vi "ToolBarcode (Get).vi"(7 "LabVIEW Web Service Request":refnum<class "Web Request.lvclass">) -> ()   [LabVIEW 2019]
uses:
  <vilib>/wsapi/Web Request.lvclass
  QDMH support files/QDMH Poly VIs/QDMH POLY Enqueue String.vi
panel:
  # "Use the Web Service Request input terminal to call the VIs on the Web Services palette. Do not remove it from the connector pane unless you don't need access to the palette."
  # "Each additional control wired to the connector pane will be available as an input in the URL. To include an indicator in terminal-mode output (the default setting), it must also be wired to the connector pane."
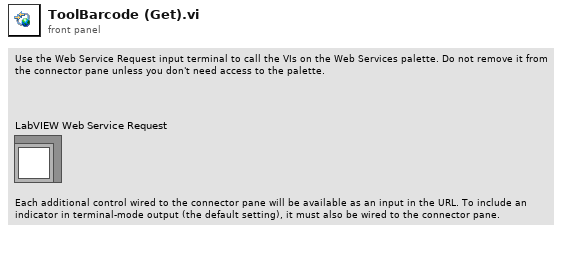
[diagram p1: front panel]
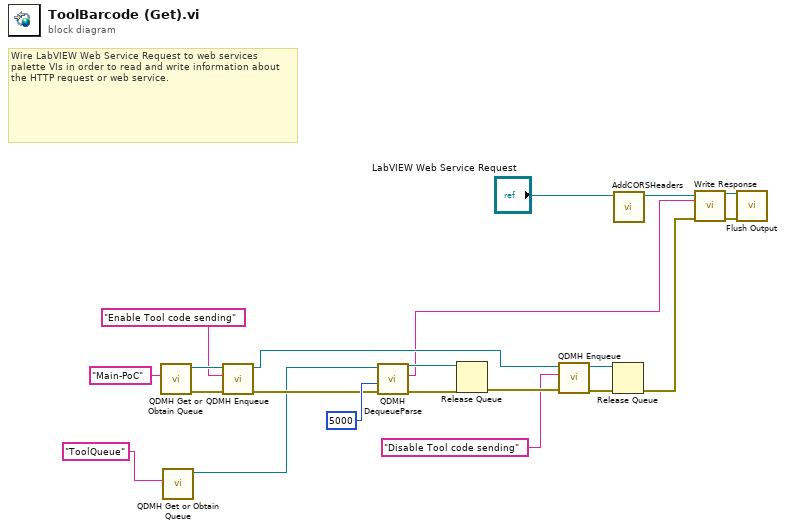
[diagram p0: block diagram]
diagram:
  # "Wire LabVIEW Web Service Request to web services palette VIs in order to read and write information about the HTTP request or web service."
  n1 = call "QDMH Get or Obtain Queue.vi"("Queue Name"="Main-PoC") -> ("error out"=w19:errorcluster, "queue out"=w20:refnum<queue>)  [unwired: 2 in, 7 out]
  n2 = call "QDMH Get or Obtain Queue.vi"("Queue Name"="ToolQueue") -> ("queue out"=w12:refnum<queue>)  [unwired: 2 in, 8 out]
  n3 = call-poly "QDMH Enqueue.vi"("error in (no error)"=w19, "State"="Enable Tool code sending", "queue"=w20) -> ("error out"=w13:errorcluster, "queue out"=w10:refnum<queue>)  [unwired: 7 out]
  n4 = call "QDMH DequeueParse.vi"("error in (no error)"=w13, "Timeout"=5000, "queue"=w12) -> ("error out"=w15:errorcluster, "State"=w2:string, "queue out"=w14:refnum<queue>)  [unwired: 5 in, 1 out]
  n5 = Release Queue(queue=w14, error in (no error)=w15) -> (error out=w11:errorcluster)  [unwired: 1 in, 2 out]
  n6 = call-poly "QDMH Enqueue.vi"("error in (no error)"=w11, "State"="Disable Tool code sending", "queue"=w10) -> ("error out"=w8:errorcluster, "queue out"=w7:refnum<queue>)  [unwired: 7 out]
  n7 = Release Queue(queue=w7, error in (no error)=w8) -> (error out=w1:errorcluster)  [unwired: 1 in, 2 out]
  n8 = call "AddCORSHeaders.vi"("Web Request in"="LabVIEW Web Service Request") -> ("Web Request out"=w4:refnum<class "Web Request.lvclass">)  [unwired: 10 in]
  n9 = call <vilib>:"Write Response.vi"("LabVIEW Web Service Request"=w4, "response string"=w2, "error in (no error)"=w1) -> ("LabVIEW Web Service Request out"=w6:refnum<class "Web Request.lvclass">, "error out"=w5:errorcluster)  [unwired: 11 in]
  n10 = call <vilib>:"Flush Output.vi"("LabVIEW Web Service Request"=w6, "error in (no error)"=w5) -> ()  [unwired: 12 in, 2 out]
